vi "Show Folder Helper.vi"(8 "Fehler (Eingang, kein Fehler)":errorcluster, 11 "Dateipfad":path) -> (0 "Fehler (Ausgang)":errorcluster)   [LabVIEW 2020, in "FTP WebDAV.lvlib"]
uses:
  FTP WebDAV.lvlib
  <vilib>/Platform/browser.llb/Open URL in Default Browser (path).vi
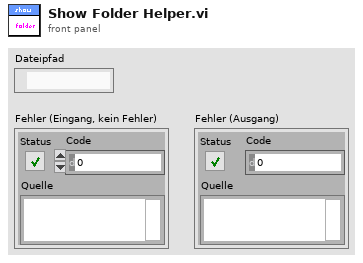
[diagram p1: front panel]
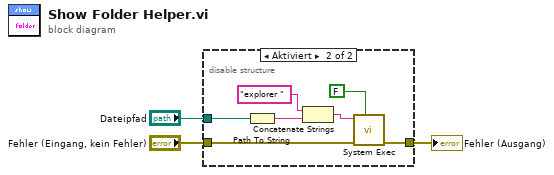
[diagram p0: block diagram]
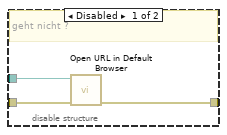
[diagram p2: hidden frame]
diagram:
  n1 = disable-structure shown="Aktiviert" {
    disable-tunnel: [w4 w10] -> w2
    disable-tunnel: "Fehler (Eingang, kein Fehler)" -> [w5 w9]
    disable-tunnel: "Dateipfad" -> [w6 w8]
    frame Disabled {
      # "geht nicht ?"
      n2 = call-poly <vilib>:"Open URL in Default Browser.vi"("error in (no error)"=w5, "path"=w6) -> ("error out"=w4:errorcluster)  [unwired: 4 in, 1 out]
    }
    frame Enabled {
      n3 = Path To String(path=w8) -> (string=w13:string)
      n4 = Concatenate Strings("explorer " ("String"), w13) -> (w11:string)
      n5 = call <vilib>:"System Exec.vi"("wait until completion? (T)"=FALSE, "error in (no error)"=w9, "command line"=w11) -> ("error out"=w10:errorcluster)  [unwired: 5 in, 3 out]
    }
  }
  "Fehler (Ausgang)" <- w2
